vi "Do.vi"(8 "error in (no error)":errorcluster, 10 "Actor in":refnum<class "Actor.lvclass">, 11 "Attribute and Convert Msg":refnum<class "Attribute and Convert Msg.lvclass">) -> (0 "error out":errorcluster, 2 "Actor out":refnum<class "Actor.lvclass">)   [LabVIEW 2012, in "Data Logger.lvlib" / "Attribute and Convert Msg.lvclass"]
doc: "This VI delivers the message to the actor by calling the appropriate method(s) on the actor."
uses:
  Attribute and Convert Msg.lvclass
  <vilib>/ActorFramework/Actor/Actor.lvclass
  Data Logger.lvclass
  Attribute and Convert Msg.lvclass/Attribute and Convert Msg.ctl
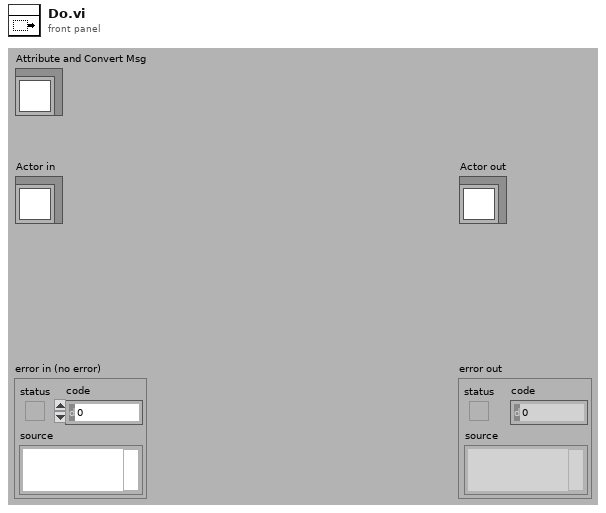
[diagram p1: front panel]
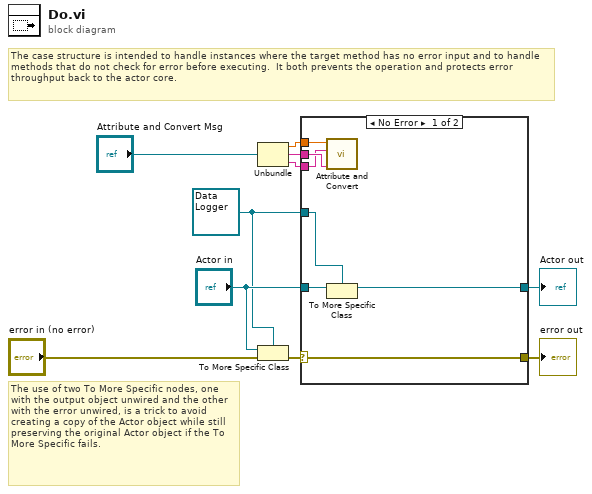
[diagram p0: block diagram]
diagram:
  w4 = refnum<class "Data Logger.lvclass"> refnum ("Actor in")
  # "The use of two To More Specific nodes, one with the output object unwired and the other with the error unwired, is a trick to avoid creating a copy of the Actor object while still preserving the original Actor object if the To More Specific fails."
  # "The case structure is intended to handle instances where the target method has no error input and to handle methods that do not check for error before executing.  It both prevents the operation and protects error throughput back to the actor core."
  n1 = Unbundle("Attribute and Convert Msg") -> (w3:dbl, w2:string, w1:string)
  n2 = To More Specific Class(target class=w4, reference="Actor in", error in="error in (no error)") -> (error out=w8:errorcluster)  [unwired: 1 out]
  n3 = case shown="No Error" w8 {
    selector: w8 -> [w17 w19]
    tunnel: [w17 w19] -> w7
    tunnel: [w14 w18] -> w6
    tunnel: "Actor in" -> [w16 w18]
    tunnel: w4 -> [w15 _]
    tunnel: w3 -> [w13 _]
    tunnel: w2 -> [w12 _]
    tunnel: w1 -> [w11 _]
    frame No Error {
      n4 = call "Attribute and Convert.vi"("Unit"=w12, "Signal Name"=w11, "Number in"=w13) -> ()  [unwired: 8 in, 1 out]
      n5 = To More Specific Class(target class=w15, reference=w16) -> (specific class reference=w14:refnum<class "Data Logger.lvclass">)  [unwired: 1 in, 1 out]
    }
    frame Error {
      # "If type check fails, pass the original object out again."
    }
  }
  "error out" <- w7
  "Actor out" <- w6
